vi "Open Pipe (reader).vi"(8 "error in (no error)":errorcluster, 11 "pathname in":string) -> (0 "error out":errorcluster, 3 "pipe reader out":refnum<data-value>)   [LabVIEW 2013, in "Linux RT IPC.lvlib" / "Pipes.lvlib" / "Unix Pipe Reader.lvclass"]
doc: "This VI creates a new writer or reader endpoint for accessing the pipe and allowing data transfer."
uses:
  Unix Pipe Reader.lvclass
  C/Controls/fcntl-linux file modes.ctl
  Unix Pipe/Unix Pipe.lvclass/Unix Pipe.ctl
  C/C.lvlib
  Unix Pipe/Unix Pipe.lvclass
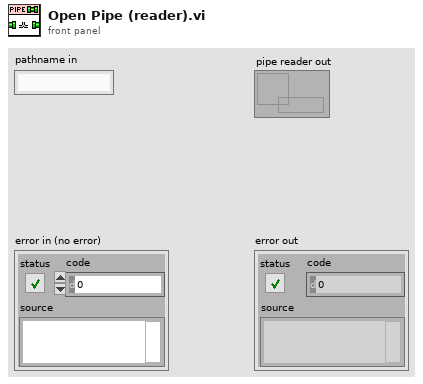
[diagram p1: front panel]
types:
  T1 = typedef "Linux RT IPC.lvlib/C.lvlib/fcntl-linux file modes.ctl" = u16
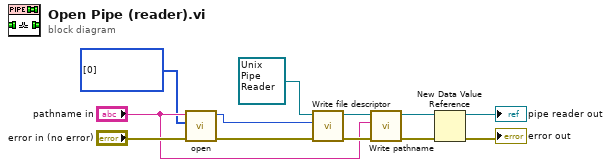
[diagram p0: block diagram]
diagram:
  w2 = T1[] [0] items=["O_RDONLY", "O_WRONLY", "O_RDWR"] ("flags")
  n1 = call "open.vi"("error in (no error)"="error in (no error)", "flags"=w2, "pathname"="pathname in") -> ("error out"=w10:errorcluster, "file descriptor"=w7:i32)  [unwired: 7 in]
  n2 = call "Write file descriptor.vi"("error in (no error)"=w10, "file descriptor"=w7, "Unix Pipe in"=refnum<class "Unix Pipe Reader.lvclass"> refnum ("Unix Pipes.lvlib:Unix Pipe Reader.lvclass")) -> ("error out"=w8:errorcluster, "Unix Pipe out"=w9:refnum<class "Unix Pipe Reader.lvclass">)  [unwired: 7 in]
  n3 = call "Write pathname.vi"("error in (no error)"=w8, "pathname"="pathname in", "Unix Pipe in"=w9) -> ("error out"=w6:errorcluster, "Unix Pipe out"=w5:refnum<class "Unix Pipe Reader.lvclass">)  [unwired: 7 in]
  n4 = New Data Value Reference(data value=w5, error in=w6) -> (data value reference=→"pipe reader out":refnum<data-value>, error out=→"error out":errorcluster)
